vi "Process Objects.vi"(9 "Read Device ID code":T1, 10 "object ID":u8, 11 "Objects":T2[](array[typedef]) {"Object ID" format="%x"}) -> (0 "object data":u8[](array[numeric]), 1 "object count":u8, 2 "next object ID":u8, 3 "more follows":u8)   [LabVIEW 2012, in "Device Data Model.lvclass"]
doc: "This VI accepts the objects of the device and the requested object information and generates the required object data and metadata."
uses:
  Device Data Model.lvclass
  Identification Parameters.ctl
  Master Function Definition/Read Device ID code.ctl
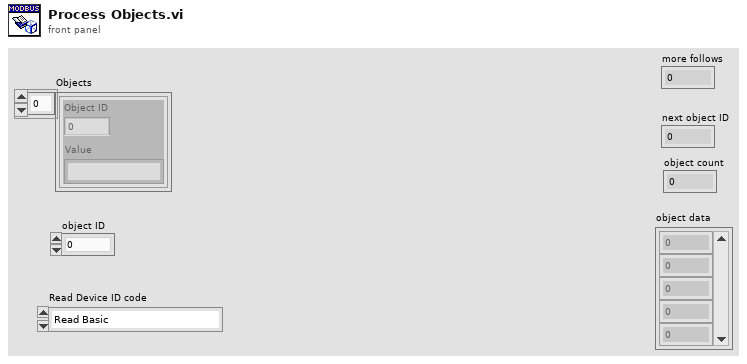
[diagram p1: front panel]
types:
  T1 = typedef "Device Data Model.lvclass/Read Device ID code.ctl" = enum8{"Read Basic", "Read Regular", "Read Extended", "Read Specific"}
  T2 = typedef "Device Data Model.lvclass/Identification Parameters.ctl" = cluster{"Object ID":u8, "Value":string}
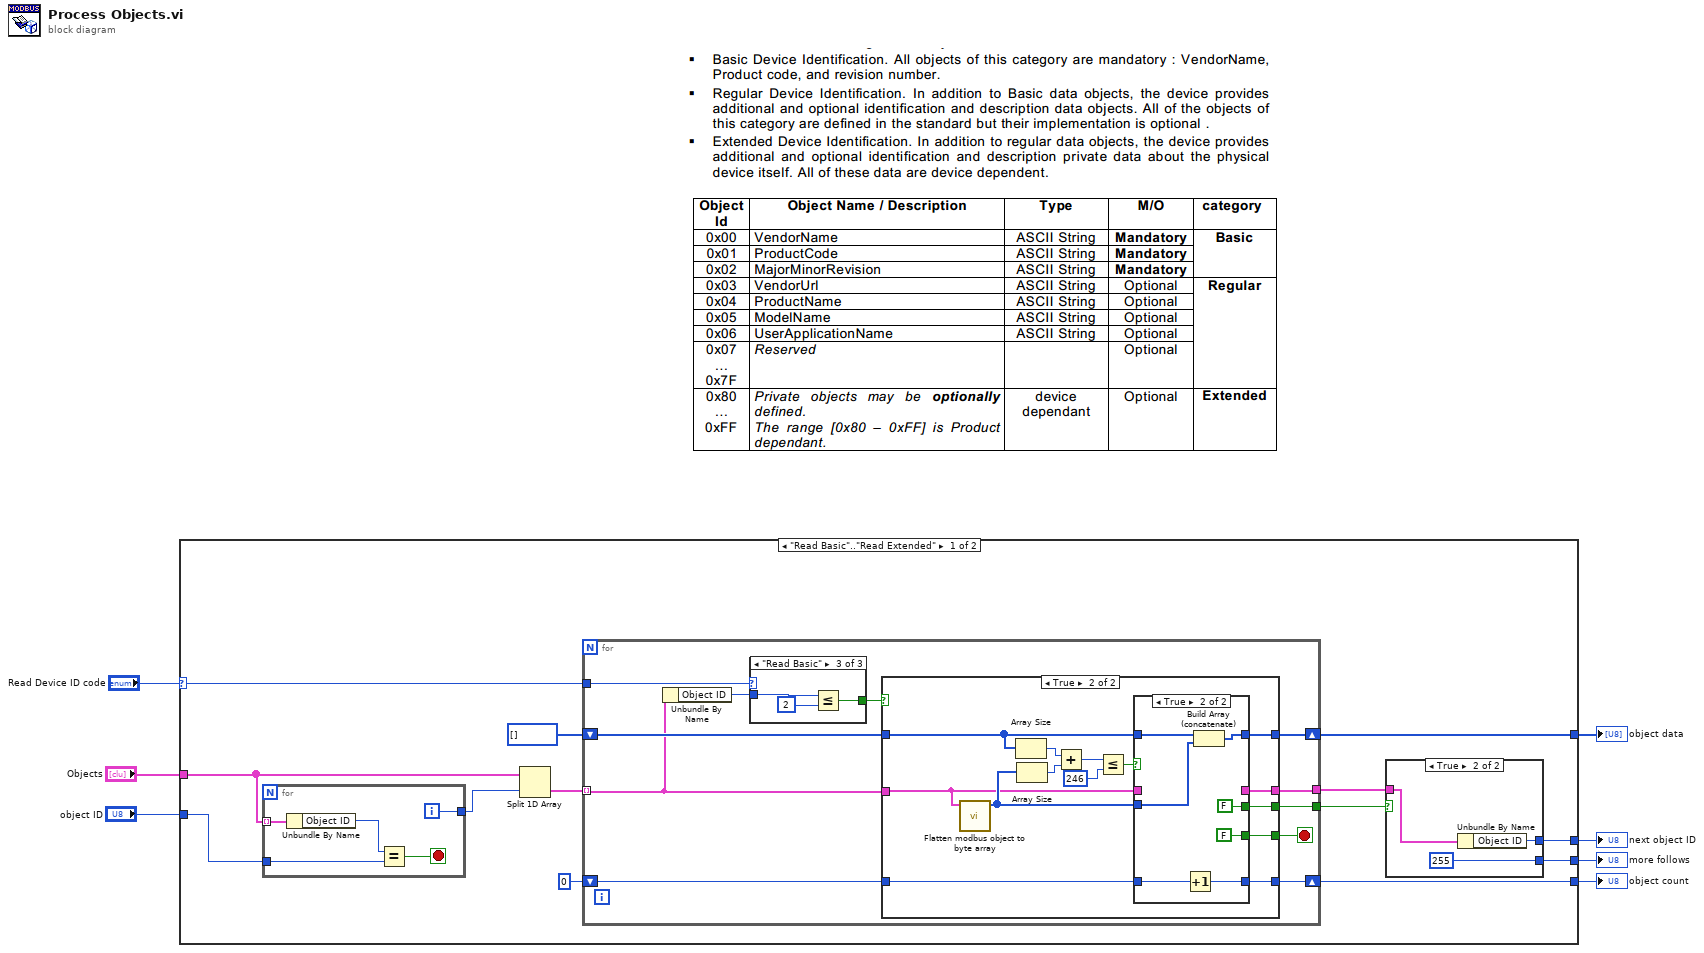
[diagram p0: block diagram]
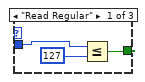
[diagram p2: hidden frame]
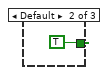
[diagram p3: hidden frame]
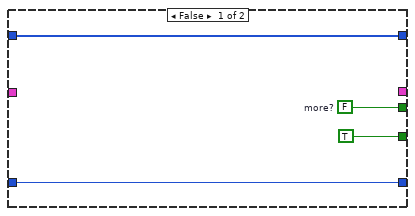
[diagram p4: hidden frame]
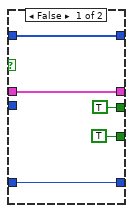
[diagram p5: hidden frame]
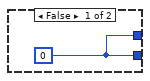
[diagram p6: hidden frame]
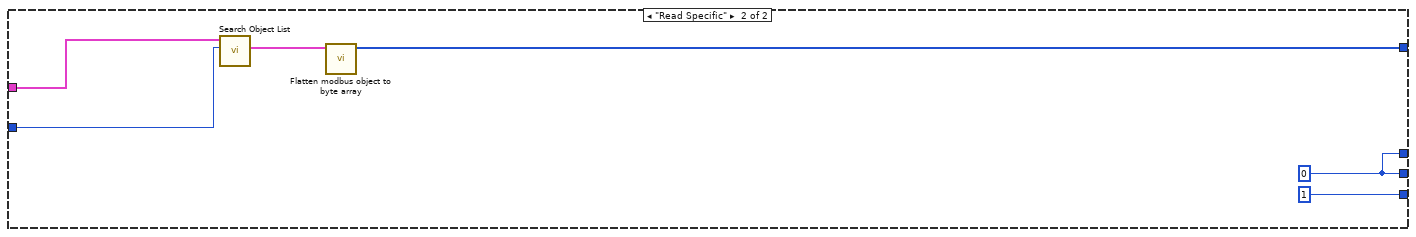
[diagram p7: hidden frame]
diagram:
  n1 = case shown="\"Read Basic\"..\"Read Extended\"" "Read Device ID code" {
    selector: "Read Device ID code" -> [w10 _]
    tunnel: "Objects" -> [w19 w83]
    tunnel: [w13 u8 1] -> w5
    tunnel: [w16 w80] -> w4
    tunnel: [w15 w80] -> w3
    tunnel: "object ID" -> [w20 w79]
    tunnel: [w11 w78] -> w1
    frame "Read Basic".."Read Extended" {
      n2 = for {
        tunnel: w19 -> [w77] mode=indexing
        tunnel: w20 -> [w76]
        tunnel: [w73] -> w18
        i -> [w73]
        stop <- w74 stop-if-true
        n3 = Unbundle By Name(w77) -> ("Object ID"=w75:u8)
        n4 = Equal?(x=w75, y=w76) -> (x = y?=w74:bool)
      }
      n5 = Split 1D Array(array=w19, index=w18) -> (second subarray=w17:T2[])  [unwired: 1 out]
      n6 = for {
        shift-right: [w28] -> w13
        shift-left: 0 -> [w29]
        shift-right: [w30] -> w11
        shift-left: u8[] [] -> [w31]
        tunnel: w17 -> [w22] mode=indexing
        tunnel: w10 -> [w27]
        tunnel: [w24] -> w9
        tunnel: [w23] -> w8
        stop <- w21 stop-if-true
        n7 = Unbundle By Name(w22) -> ("Object ID"=w26:u8)
        n8 = case shown="\"Read Basic\"" w27 {
          tunnel: w26 -> [w34 _ w38]
          tunnel: [w32 TRUE w36] -> w25
          frame "Read Regular" {
            n9 = Less Or Equal?(x=w34, y=u8 127) -> (x <= y?=w32:bool)
          }
          frame Default {
          }
          frame "Read Basic" {
            n10 = Less Or Equal?(x=w38, y=u8 2) -> (x <= y?=w36:bool)
          }
        }
        n11 = case shown="True" w25 {
          tunnel: w31 -> [w41 w50]
          tunnel: [w41 w49] -> w30
          tunnel: w29 -> [w40 w48]
          tunnel: [w40 w47] -> w28
          tunnel: [TRUE w46] -> w21
          tunnel: w22 -> [_ w45]
          tunnel: [w39 w43] -> w24
          tunnel: [_ w44] -> w23
          frame False {
            w39 = FALSE  # more?
          }
          frame True {
            n12 = call "Flatten modbus object to byte array.vi"("Object"=w45) -> ("byte array"=w51:u8[])  [unwired: 10 in]
            n13 = Array Size(array=w50) -> (size(s)=w55:i32)
            n14 = Array Size(array=w51) -> (size(s)=w56:i32)
            n15 = Add(x=w55, y=w56) -> (x+y=w54:i32)
            n16 = Less Or Equal?(x=w54, y=246) -> (x <= y?=w52:bool)
            n17 = case shown="True" w52 {
              tunnel: w51 -> [_ w66]
              tunnel: w50 -> [w60 w68]
              tunnel: [w60 w67] -> w49
              tunnel: w48 -> [w61 w65]
              tunnel: [w61 w64] -> w47
              tunnel: [TRUE FALSE] -> w46
              tunnel: w45 -> [w58 _]
              tunnel: [w58 _] -> w44
              tunnel: [TRUE FALSE] -> w43
              frame False {
              }
              frame True {
                n18 = Increment(x=w65) -> (x+1=w64:i32)
                n19 = Build Array (concatenate)(w68, w66) -> (w67:u8[])
              }
            }
          }
        }
      }
      n20 = case shown="True" w9 {
        tunnel: [w69 u8 255] -> w16
        tunnel: [w69 w70] -> w15
        tunnel: w8 -> [_ w71]
        frame False {
          w69 = u8 0
        }
        frame True {
          n21 = Unbundle By Name(w71) -> ("Object ID"=w70:u8)
        }
      }
    }
    frame "Read Specific" {
      w80 = u8 0
      n22 = call "Search Object List.vi"("Object ID"=w79, "Objects"=w83) -> ("Object"=w82:T2)  [unwired: 7 in, 2 out]
      n23 = call "Flatten modbus object to byte array.vi"("Object"=w82) -> ("byte array"=w78:u8[])  [unwired: 10 in]
    }
  }
  "object data" <- w1
  "next object ID" <- w3
  "more follows" <- w4
  "object count" <- w5
